vi "Stop Sequence.vi"(8 "error in (no error)":errorcluster, 11 "POLARIS Target Focus Actor in":refnum<class "POLARIS Target Focus Actor.lvclass">) -> (0 "error out":errorcluster, 3 "POLARIS Target Focus Actor out":refnum<class "POLARIS Target Focus Actor.lvclass">)   [LabVIEW 2014, in "POLARIS Target Focus Actor.lvlib" / "POLARIS Target Focus Actor.lvclass"]
uses:
  POLARIS Target Focus Actor.lvclass
  POLARIS Target Focus Actor.lvclass/POLARIS Target Focus Actor.ctl
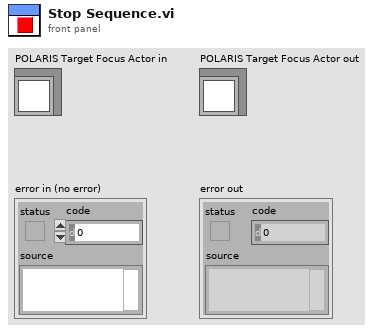
[diagram p1: front panel]
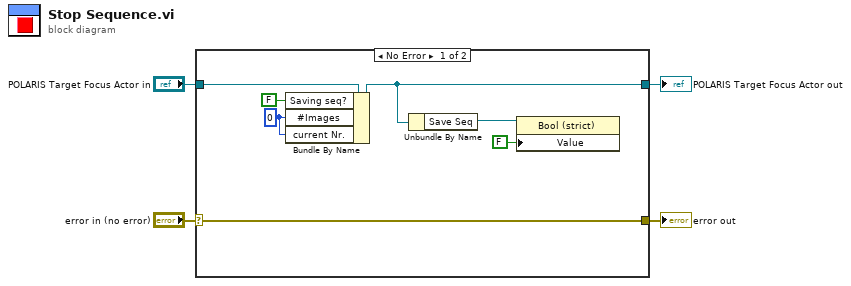
[diagram p0: block diagram]
diagram:
  n1 = case shown="No Error" "error in (no error)" {
    selector: "error in (no error)" -> [w10 w13]
    tunnel: [w10 w13] -> w3
    tunnel: [w8 w12] -> w1
    tunnel: "POLARIS Target Focus Actor in" -> [w11 w12]
    frame No Error {
      w5 = u16 0 ("#Images")
      n2 = Bundle By Name(cluster=w11, "Saving seq?"=FALSE, "#Images"=w5, "current Nr."=w5) -> (w8:refnum<class "POLARIS Target Focus Actor.lvclass">)
      n3 = Unbundle By Name(w8) -> ("Save Seq"=w7:refnum<vi>)
      n4 = property class="Bool (strict)"(reference=w7, "Value"=FALSE) -> ()  [unwired: 1 in, 2 out]
    }
    frame Error {
    }
  }
  "error out" <- w3
  "POLARIS Target Focus Actor out" <- w1
